vi "main_analyzer.vi"(8 "error in (no error)":errorcluster) -> (0 "error out":errorcluster)   [LabVIEW 2020]
uses:
  #typedefs/#typedef_cluster_ANALYZE_Options.ctl
  #typedefs/#typedef_enum_QueueActions.ctl
  #typedefs/#typedef_cluster_ANALYZE_QueueData.ctl
  #typedefs/#typedef_enum_ANALYZE_States.ctl
  #typedefs/#typedef_enum_EventActions.ctl
  #typedefs/#typedef_cluster_ANALYZE_Data.ctl
  <vilib>/vision/Image Controls.llb/IMAQ Image.ctl
  #typedefs/#typedef_cluster_CTRL_QueueData.ctl
  #typedefs/#typedef_enum_CTRL_States.ctl
panel:
  in  "Save Button":bool
  in  "Analyze Options":T1
  out "Image":T2(plugin-control)
  in  "Process Button":bool
  in  "Exit Button":bool
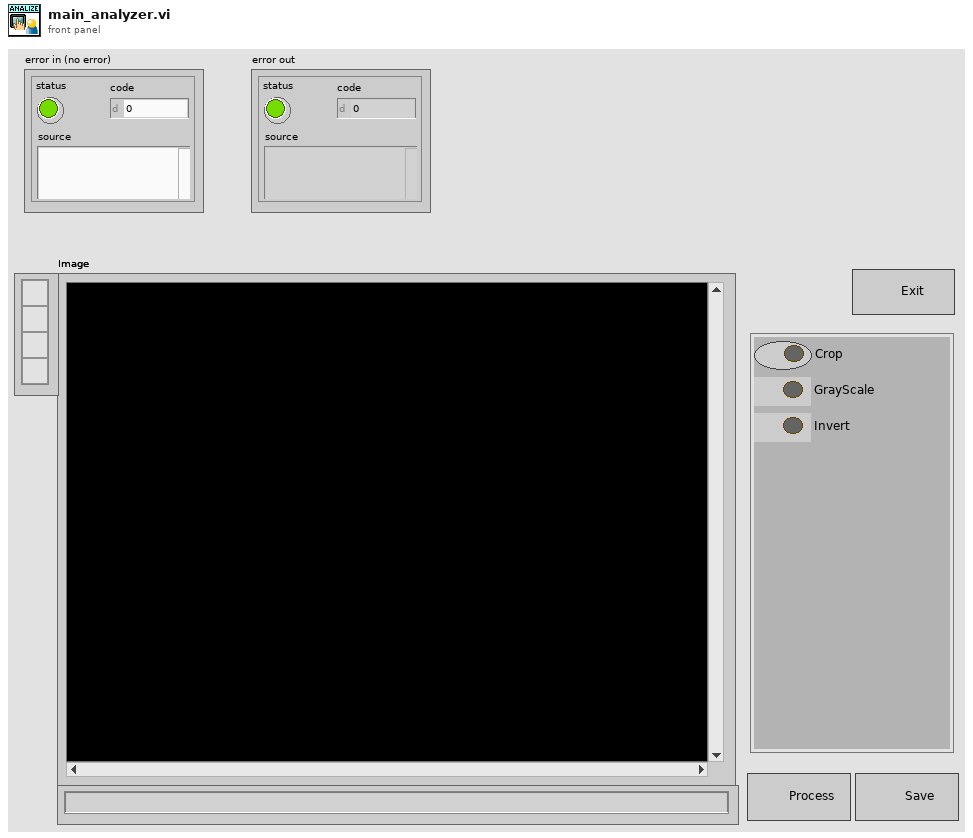
[diagram p1: front panel]
types:
  T1 = typedef "#typedef_cluster_ANALYZE_Options.ctl" = cluster{"Crop":bool, "GrayScale":bool, "Invert":bool}
  T2 = typedef "IMAQ Image.ctl" = refnum<image>
  T3 = typedef "#typedef_enum_EventActions.ctl" = enum16{"Obtain", "GetRef", "Generate", "Destroy"}
  T4 = typedef "#typedef_cluster_ANALYZE_QueueData.ctl" = cluster{"Cmd":T5, "Variant":variant}
  T5 = typedef "#typedef_enum_ANALYZE_States.ctl" = enum16{"Init", "Open", "UpdateOptions", "Process", "Save", "ErrorHandling", "ExitRequest", "Exit"}
  T6 = typedef "#typedef_enum_QueueActions.ctl" = enum16{"Obtain", "GetRef", "Enqueue", "Release"}
  T7 = enum32{"Invalid", "Standard", "Closed", "Hidden", "Minimized", "Maximized"}
  T8 = typedef "#typedef_enum_CTRL_States.ctl" = enum16{"Init", "AnalyzeImage", "SaveImage", "ErrorHandling", "ExitRequest", "Exit"}
  T9 = typedef "#typedef_cluster_CTRL_QueueData.ctl" = cluster{"Cmd":T8, "Variant":variant}
  T10 = typedef "#typedef_cluster_ANALYZE_Data.ctl" = cluster{"Image":T2, "Options":T1}
  T11 = cluster{"Global Rectangle":i32[], "Contours":cluster{"Contour Type":u32, "ROI Type":u32, "Points":i32[]}[]}
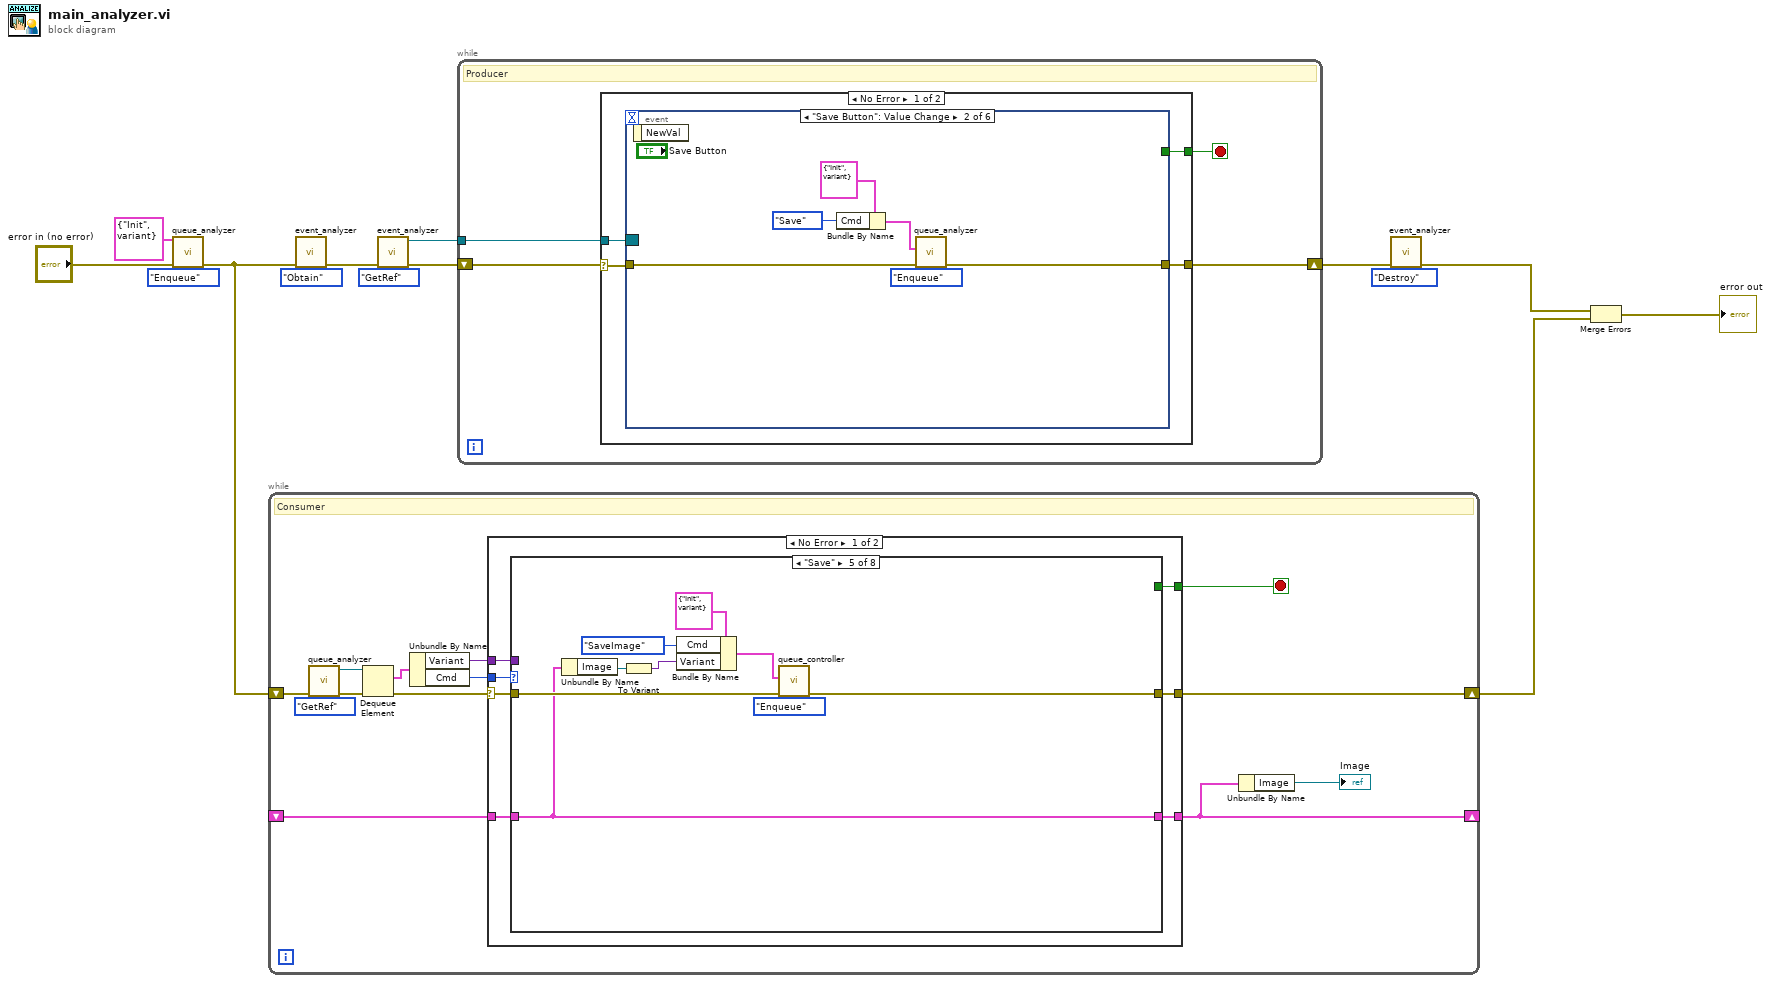
[diagram p0: block diagram]
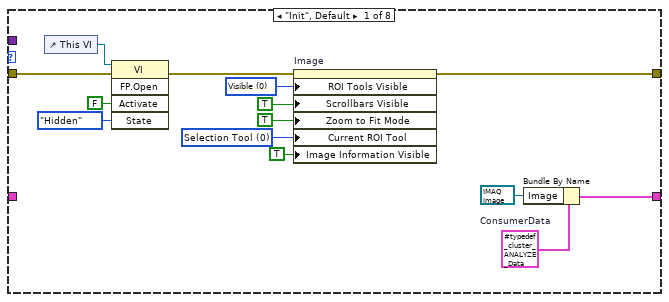
[diagram p2: hidden frame]
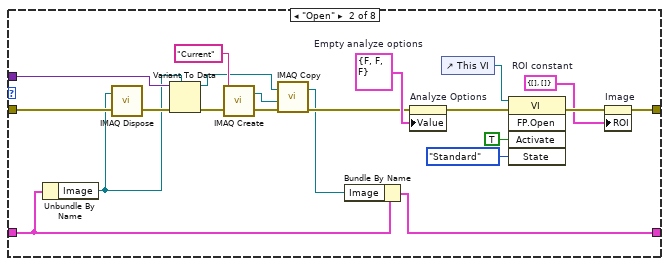
[diagram p3: hidden frame]
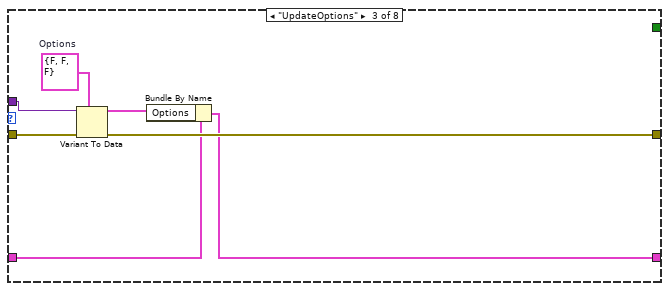
[diagram p4: hidden frame]
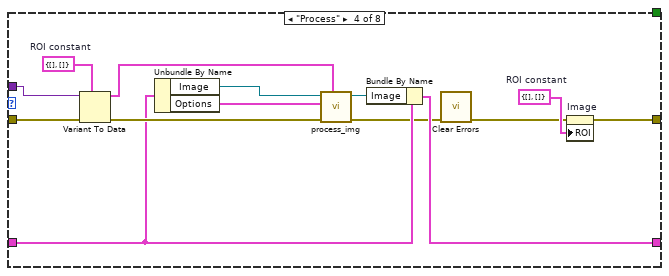
[diagram p5: hidden frame]
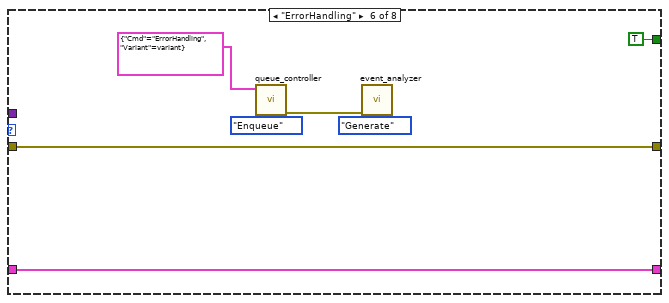
[diagram p6: hidden frame]
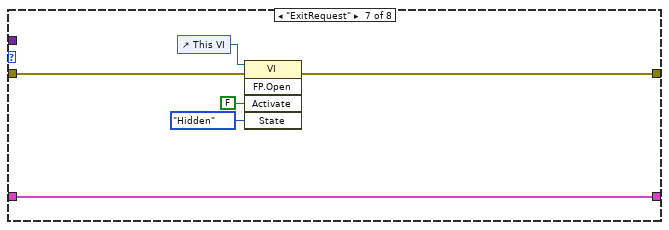
[diagram p7: hidden frame]
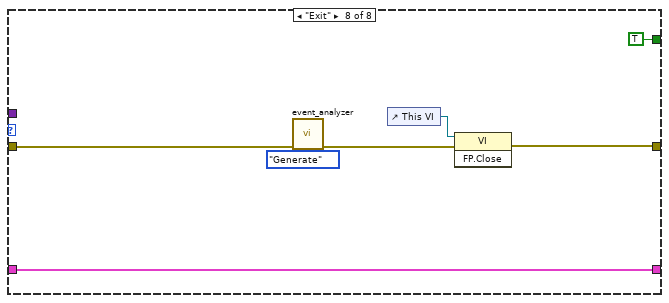
[diagram p8: hidden frame]
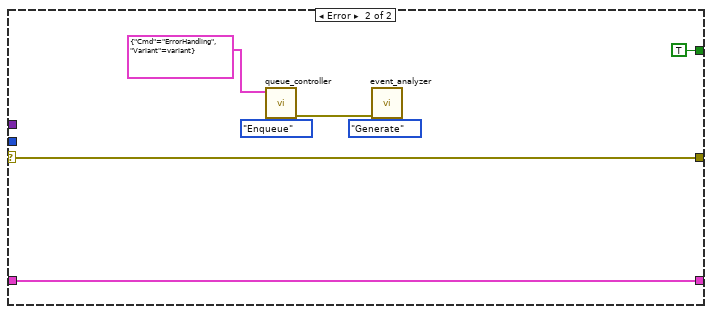
[diagram p9: hidden frame]
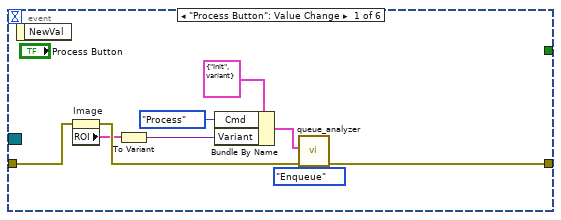
[diagram p10: hidden frame]
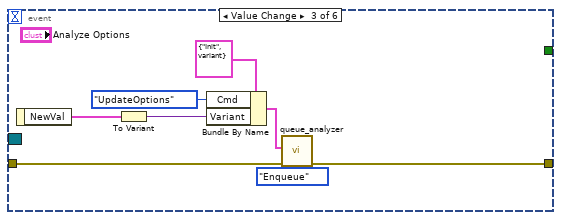
[diagram p11: hidden frame]
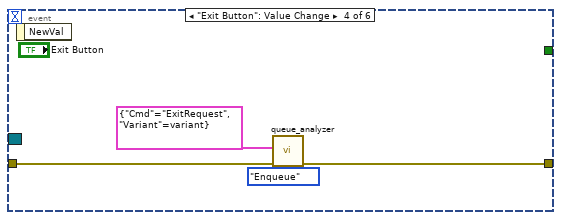
[diagram p12: hidden frame]
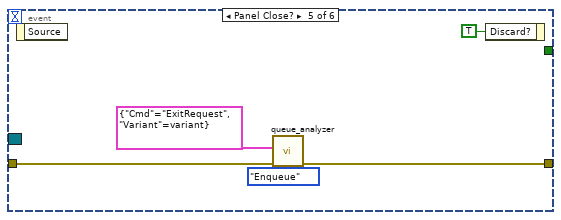
[diagram p13: hidden frame]
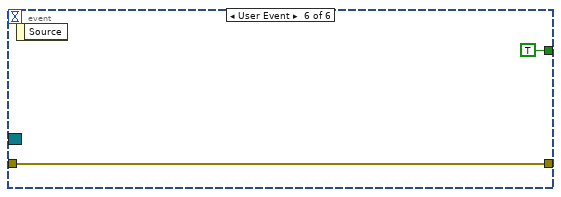
[diagram p14: hidden frame]
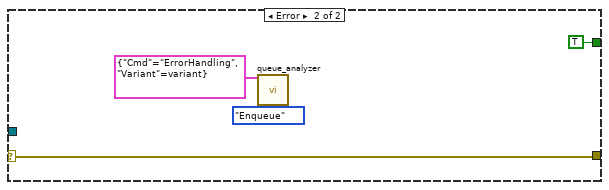
[diagram p15: hidden frame]
diagram:
  n1 = call "queue_analyzer.vi"("QueueActions"=#typedef_enum_QueueActions."Enqueue", "error in (no error)"="error in (no error)", "QueueDataIn"=T4 {"Cmd"=enum."Init", "Variant"=variant}) -> ("error out"=w5:errorcluster)  [unwired: 7 in, 1 out]
  n2 = while {
    shift-right: [w16] -> w14
    shift-left: w5 -> [w24]
    shift-right: [w18] -> _
    shift-left: _ -> [w19]
    stop <- w25 stop-if-true
    # "Consumer"
    n3 = call "queue_analyzer.vi"("QueueActions"=#typedef_enum_QueueActions."GetRef", "error in (no error)"=w24) -> ("error out"=w23:errorcluster, "queue out"=w22:refnum<queue>)  [unwired: 8 in]
    n4 = Dequeue Element(queue=w22, error in (no error)=w23) -> (element=w27:T4, error out=w15:errorcluster)  [unwired: 1 in, 2 out]
    n5 = Unbundle By Name(w27) -> ("Variant"=w21:variant, "Cmd"=w26:T5)
    n6 = case shown="No Error" w15 {
      selector: w15 -> [w28 w125]
      tunnel: w26 -> [w34 _]
      tunnel: [w33 TRUE] -> w25
      tunnel: w21 -> [w32 _]
      tunnel: w19 -> [w31 w124]
      tunnel: [w30 w124] -> w18
      tunnel: [w29 w125] -> w16
      frame No Error {
        n7 = case shown="\"Save\"" w34 {
          tunnel: w28 -> [w41 w58 w74 w90 w99 w106 w111 w119]
          tunnel: [w48 w62 w73 w83 w98 w106 w110 w113] -> w29
          tunnel: [_ _ _ _ _ TRUE _ TRUE] -> w33
          tunnel: w32 -> [_ w66 w75 w89 _ _ _ _]
          tunnel: [w35 w64 w70 w84 w93 w105 w107 w116] -> w30
          tunnel: w31 -> [_ w65 w72 w86 w93 w105 w107 w116]
          frame "Init", Default {
            w37 = T10 {"Image"=refnum, "Options"={"Crop"=FALSE, "GrayScale"=FALSE, "Invert"=FALSE}}  # ConsumerData
            w44 = u32 0 items=["Zoom Tool"=8, "Selection Tool"=0, "Pan Tool"=9, "Point Tool"=1, "Line Tool"=2, "Rectangle Tool"=3, "Rotated Rectangle Tool"=12, "Polyline Tool"=10, "Polygon Tool"=5, "Freehand Tool"=11, "Closed Freehand Tool"=6, "Ellipse Tool"=4, "Annulus Tool"=7] ("Current ROI Tool")
            w47 = u32 0 items=["Visible", "Hidden", "Hidden, Use WindTools Palette"] ("ROI Tools Visible")
            n8 = control-ref of="This VI"() -> (w42:refnum<vi>)
            n9 = invoke class="VI" method="FP.Open"(reference=w42, error in=w41, "Activate"=FALSE ("Activate?"), "State"=T7."Hidden") -> (error out=w40:errorcluster)  [unwired: 1 in, 4 out]
            n10 = property on="Image" class="ImageControl"(error in=w40, "ROI Tools Visible"=w47, "Scrollbars Visible"=TRUE, "Zoom to Fit Mode"=TRUE, "Current ROI Tool"=w44, "Image Information Visible"=TRUE) -> (error out=w48:errorcluster)  [unwired: 1 in, 1 out]
            n11 = Bundle By Name(cluster=w37, "Image"=T2 refnum) -> (w35:T10)
          }
          frame "Open" {
            w59 = T1 {"Crop"=FALSE, "GrayScale"=FALSE, "Invert"=FALSE}  # Empty analyze options
            w61 = T11 {"Global Rectangle"=[], "Contours"=[]}  # ROI constant
            n12 = Unbundle By Name(w65) -> ("Image"=w56:T2)
            n13 = call "IMAQ Dispose"("Image"=w56, "error in (no error)"=w58) -> ("error out"=w57:errorcluster)  [unwired: 4 in]
            n14 = Variant To Data(error in=w57, type=w56, Variant=w66) -> (data=w50:T2, error out=w55:errorcluster)
            n15 = call "IMAQ Create"("Image Name"="Current", "error in (no error)"=w55) -> ("New Image"=w51:T2, "error out"=w53:errorcluster)  [unwired: 3 in]
            n16 = call "IMAQ Copy"("error in (no error)"=w53, "Image Dst"=w51, "Image Src"=w50) -> ("error out"=w52:errorcluster, "Image Dst Out"=w49:T2)  [unwired: 3 in]
            n17 = Bundle By Name(cluster=w65, "Image"=w49) -> (w64:T10)
            n18 = property on="Analyze Options" class="Clust (strict)"(error in=w52, "Value"=w59) -> (error out=w60:errorcluster)  [unwired: 1 in, 1 out]
            n19 = control-ref of="This VI"() -> (w69:refnum<vi>)
            n20 = invoke class="VI" method="FP.Open"(reference=w69, error in=w60, "Activate"=TRUE ("Activate?"), "State"=T7."Standard") -> (error out=w63:errorcluster)  [unwired: 1 in, 4 out]
            n21 = property on="Image" class="ImageControl"(error in=w63, "ROI"=w61) -> (error out=w62:errorcluster)  [unwired: 1 in, 1 out]
          }
          frame "UpdateOptions" {
            w76 = T1 {"Crop"=FALSE, "GrayScale"=FALSE, "Invert"=FALSE}  # Options
            n22 = Variant To Data(error in=w74, type=w76, Variant=w75) -> (data=w71:T1, error out=w73:errorcluster)
            n23 = Bundle By Name(cluster=w72, "Options"=w71) -> (w70:T10)
          }
          frame "Process" {
            w82 = T11 {"Global Rectangle"=[], "Contours"=[]}  # ROI constant
            w80 = T11 {"Global Rectangle"=[], "Contours"=[]}  # ROI constant
            n24 = Variant To Data(error in=w90, type=w80, Variant=w89) -> (data=w79:T11, error out=w88:errorcluster)
            n25 = Unbundle By Name(w86) -> ("Image"=w87:T2, "Options"=w81:T1)
            n26 = call "process_img.vi"("ROI"=w79, "error in (no error)"=w88, "Options"=w81, "Image Src"=w87) -> ("error out"=w78:errorcluster, "Image Dst"=w85:T2)  [unwired: 6 in]
            n27 = Bundle By Name(cluster=w86, "Image"=w85) -> (w84:T10)
            n28 = call <vilib>:"Clear Errors.vi"("error in (no error)"=w78) -> ("error out"=w77:errorcluster)  [unwired: 5 in, 1 out]
            n29 = property on="Image" class="ImageControl"(error in=w77, "ROI"=w82) -> (error out=w83:errorcluster)  [unwired: 1 in, 1 out]
          }
          frame "Save" {
            n30 = Unbundle By Name(w93) -> ("Image"=w92:T2)
            n31 = To Variant(anything=w92) -> (Variant=w91:variant)
            n32 = Bundle By Name(cluster=T9 {"Cmd"=enum."Init", "Variant"=variant} ("QueueDataIn"), "Cmd"=#typedef_enum_CTRL_States."SaveImage", "Variant"=w91) -> (w94:T9)
            n33 = call "queue_controller.vi"("QueueActions"=#typedef_enum_QueueActions."Enqueue", "error in (no error)"=w99, "QueueDataIn"=w94) -> ("error out"=w98:errorcluster)  [unwired: 7 in, 1 out]
          }
          frame "ErrorHandling" {
            n34 = call "queue_controller.vi"("QueueActions"=#typedef_enum_QueueActions."Enqueue", "QueueDataIn"=T9 {"Cmd"=enum."ErrorHandling", "Variant"=variant}) -> ("error out"=w100:errorcluster)  [unwired: 8 in, 1 out]
            n35 = call "event_analyzer.vi"("EventAction"=#typedef_enum_EventActions."Generate", "error in (no error)"=w100) -> ()  [unwired: 8 in, 2 out]
          }
          frame "ExitRequest" {
            n36 = control-ref of="This VI"() -> (w112:refnum<vi>)
            n37 = invoke class="VI" method="FP.Open"(reference=w112, error in=w111, "Activate"=FALSE ("Activate?"), "State"=T7."Hidden") -> (error out=w110:errorcluster)  [unwired: 1 in, 4 out]
          }
          frame "Exit" {
            n38 = call "event_analyzer.vi"("EventAction"=#typedef_enum_EventActions."Generate", "error in (no error)"=w119) -> ("error out"=w114:errorcluster)  [unwired: 8 in, 1 out]
            n39 = control-ref of="This VI"() -> (w115:refnum<vi>)
            n40 = invoke class="VI" method="FP.Close"(reference=w115, error in=w114) -> (error out=w113:errorcluster)  [unwired: 1 in, 2 out]
          }
        }
      }
      frame Error {
        n41 = call "queue_controller.vi"("QueueActions"=#typedef_enum_QueueActions."Enqueue", "QueueDataIn"=T9 {"Cmd"=enum."ErrorHandling", "Variant"=variant}) -> ("error out"=w120:errorcluster)  [unwired: 8 in, 1 out]
        n42 = call "event_analyzer.vi"("EventAction"=#typedef_enum_EventActions."Generate", "error in (no error)"=w120) -> ()  [unwired: 8 in, 2 out]
      }
    }
    n43 = Unbundle By Name(w18) -> ("Image"=→"Image":T2)
  }
  n44 = call "event_analyzer.vi"("EventAction"=#typedef_enum_EventActions."Obtain", "error in (no error)"=w5) -> ("error out"=w6:errorcluster)  [unwired: 8 in, 1 out]
  n45 = call "event_analyzer.vi"("EventAction"=#typedef_enum_EventActions."GetRef", "error in (no error)"=w6) -> ("error out"=w8:errorcluster, "Event Registration Refnum"=w7:refnum<event-registration>)  [unwired: 8 in]
  n46 = while {
    tunnel: w7 -> [w128]
    shift-right: [w129] -> w4
    shift-left: w8 -> [w127]
    stop <- w130 stop-if-true
    # "Producer"
    n47 = case shown="No Error" w127 {
      selector: w127 -> [w131 w171]
      tunnel: [w134 TRUE] -> w130
      tunnel: [w133 w171] -> w129
      tunnel: w128 -> [w132 _]
      frame No Error {
        n48 = event shown="[1] \"Save Button\": Value Change" {
          selector: w132 -> [_ _ _ _ _ _]
          dyn-events: _ -> [_ _ _ _ _ _]
          timeout: _ -> [_ _ _ _ _ _]
          tunnel: [_ _ _ _ _ TRUE] -> w134
          tunnel: w131 -> [w138 w144 w156 w160 w165 w168]
          tunnel: [w143 w149 w155 w159 w164 w168] -> w133
          event "Process Button": Value Change {
            n49 = event-data() -> ()  [unwired: 1 in, 1 out]
            n50 = property on="Image" class="ImageControl"(error in=w138) -> (error out=w137:errorcluster, "ROI"=w136:T11)  [unwired: 1 in, 1 out]
            n51 = To Variant(anything=w136) -> (Variant=w135:variant)
            n52 = Bundle By Name(cluster=T4 {"Cmd"=enum."Init", "Variant"=variant} ("QueueDataIn"), "Cmd"=#typedef_enum_ANALYZE_States."Process", "Variant"=w135) -> (w139:T4)
            n53 = call "queue_analyzer.vi"("QueueActions"=#typedef_enum_QueueActions."Enqueue", "error in (no error)"=w137, "QueueDataIn"=w139) -> ("error out"=w143:errorcluster)  [unwired: 7 in, 1 out]
          }
          event "Save Button": Value Change {
            n54 = event-data() -> ()  [unwired: 1 in, 1 out]
            n55 = Bundle By Name(cluster=T4 {"Cmd"=enum."Init", "Variant"=variant} ("QueueDataIn"), "Cmd"=#typedef_enum_ANALYZE_States."Save") -> (w145:T4)
            n56 = call "queue_analyzer.vi"("QueueActions"=#typedef_enum_QueueActions."Enqueue", "error in (no error)"=w144, "QueueDataIn"=w145) -> ("error out"=w149:errorcluster)  [unwired: 7 in, 1 out]
          }
          event Value Change {
            n57 = event-data() -> ("NewVal"=w151:T1)  [unwired: 1 in]
            n58 = To Variant(anything=w151) -> (Variant=w150:variant)
            n59 = Bundle By Name(cluster=T4 {"Cmd"=enum."Init", "Variant"=variant} ("QueueDataIn"), "Cmd"=#typedef_enum_ANALYZE_States."UpdateOptions", "Variant"=w150) -> (w153:T4)
            n60 = call "queue_analyzer.vi"("QueueActions"=#typedef_enum_QueueActions."Enqueue", "error in (no error)"=w156, "QueueDataIn"=w153) -> ("error out"=w155:errorcluster)  [unwired: 7 in, 1 out]
          }
          event "Exit Button": Value Change {
            n61 = event-data() -> ()  [unwired: 1 in, 1 out]
            n62 = call "queue_analyzer.vi"("QueueActions"=#typedef_enum_QueueActions."Enqueue", "error in (no error)"=w160, "QueueDataIn"=T4 {"Cmd"=enum."ExitRequest", "Variant"=variant}) -> ("error out"=w159:errorcluster)  [unwired: 7 in, 1 out]
          }
          event Panel Close? {
            n63 = event-data() -> ()  [unwired: 1 in, 1 out]
            n64 = call "queue_analyzer.vi"("QueueActions"=#typedef_enum_QueueActions."Enqueue", "error in (no error)"=w165, "QueueDataIn"=T4 {"Cmd"=enum."ExitRequest", "Variant"=variant}) -> ("error out"=w164:errorcluster)  [unwired: 7 in, 1 out]
            n65 = event-data("Discard?"=TRUE) -> ()  [unwired: 1 in, 1 out]
          }
          event User Event {
            n66 = event-data() -> ()  [unwired: 1 in, 1 out]
          }
        }
      }
      frame Error {
        n67 = call "queue_analyzer.vi"("QueueActions"=#typedef_enum_QueueActions."Enqueue", "QueueDataIn"=T4 {"Cmd"=enum."ErrorHandling", "Variant"=variant}) -> ()  [unwired: 8 in, 2 out]
      }
    }
  }
  n68 = call "event_analyzer.vi"("EventAction"=#typedef_enum_EventActions."Destroy", "error in (no error)"=w4) -> ("error out"=w3:errorcluster)  [unwired: 8 in, 1 out]
  n69 = Merge Errors(w3, w14) -> (→"error out":errorcluster)
